vi "svx_SC Line Plot Line Style Write.vi"(4 "error in (no error)":errorcluster, 5 "Value":u8, 6 "Container State":T5, 7 "Display State In":T1={"X Scale"={"Name"="Horizontal", "format string"="%#.2g", "Major Color"=16777238, "Minor Color"=16777216, "Scale Visible"=TRUE, " Label Visible"=TRUE, "Grid Style"=1, "Maximum"=1.0, "Minimum"=-1.0}, "Y Scale"={"Name"="Vertical", "format string"="%#.2g", "Major Color"=16777238, "Minor Color"=16777216, "Scale Visible"=TRUE, " Label Visible"=TRUE, "Grid Style"=1, "Maximum"=1.0, "Minimum"=-1.0}, "Plot"={"Point Style"=0, "Line Width"=0, "Line Style"=0, "Plot Color"=16860, "Point/fill"=16860}, "Arrow Color"=16860, "Autoscale"=TRUE, "Property Name"=[], "Container Bounds"={"Width"=550, "Height"=313}, "Background color"=16777226, "Annotation List"=[], "Cursor"={"Cursor Point Style"=13, "Cursor Style"=4, "Cursor Line Width"=1, "Cursor Line Style"=0, "Cursor Color"=16711680, "Cursor Name Visible"=TRUE, "Cursor Visible"=TRUE, "Cursor Position"={"X"=0.0, "Y"=0.0}, "Cursor Index"=0, "Lock Cursor Name"=FALSE, "Cursor reference"=0.0}, "size"=0, "Boundary Color"=9868950, "Maximum"=1.0, "Marker Point Style"=2, "Maker Visible"=TRUE, "Marker Color"=16860, "pair strings []"=[], "clearance boundary"=[{"boundary"={"x axis"=0.0, "y axis"=0.0}, "start point"=enum."center"}], "Custom pair name"=FALSE, "selector.visible"=TRUE, "Cursor Release"=refnum, "Children Tags"=[], "open?"=TRUE, "pair index"=[], "Legend Width"=200, " Parents Tags"="", "Label"="", "Legend Background"=16777226, "Legend Font"=16777222, "scale fit"=2, "user strings []"=[], "Item Width"=0, "out of state queue"=refnum, "property nodes"=refnum, "Kind"=enum."X-Scale", "Scale Range Change"=refnum} {"pair index" min=0}) -> (0 "error out":errorcluster, 3 "Display State Out":T1={"X Scale"={"Name"="Horizontal", "format string"="%#.2g", "Major Color"=16777238, "Minor Color"=16777216, "Scale Visible"=TRUE, " Label Visible"=TRUE, "Grid Style"=1, "Maximum"=1.0, "Minimum"=-1.0}, "Y Scale"={"Name"="Vertical", "format string"="%#.2g", "Major Color"=16777238, "Minor Color"=16777216, "Scale Visible"=TRUE, " Label Visible"=TRUE, "Grid Style"=1, "Maximum"=1.0, "Minimum"=-1.0}, "Plot"={"Point Style"=0, "Line Width"=0, "Line Style"=0, "Plot Color"=16860, "Point/fill"=16860}, "Arrow Color"=16860, "Autoscale"=TRUE, "Property Name"=[], "Container Bounds"={"Width"=550, "Height"=313}, "Background color"=16777226, "Annotation List"=[], "Cursor"={"Cursor Point Style"=13, "Cursor Style"=4, "Cursor Line Width"=1, "Cursor Line Style"=0, "Cursor Color"=16711680, "Cursor Name Visible"=TRUE, "Cursor Visible"=TRUE, "Cursor Position"={"X"=0.0, "Y"=0.0}, "Cursor Index"=0, "Lock Cursor Name"=FALSE, "Cursor reference"=0.0}, "size"=0, "Boundary Color"=9868950, "Maximum"=1.0, "Marker Point Style"=2, "Maker Visible"=TRUE, "Marker Color"=16860, "pair strings []"=[], "clearance boundary"=[{"boundary"={"x axis"=0.0, "y axis"=0.0}, "start point"=enum."center"}], "Custom pair name"=FALSE, "selector.visible"=TRUE, "Cursor Release"=refnum, "Children Tags"=[], "open?"=TRUE, "pair index"=[], "Legend Width"=200, " Parents Tags"="", "Label"="", "Legend Background"=16777226, "Legend Font"=16777222, "scale fit"=2, "user strings []"=[], "Item Width"=0, "out of state queue"=refnum, "property nodes"=refnum, "Kind"=enum."X-Scale", "Scale Range Change"=refnum} {"pair index" min=0})   [LabVIEW 2017, in "SVX SC Line.xctl"]
uses:
  <vilib>/addons/_XControls/Shaft Centerline/SVX SC Line.xctl
  <vilib>/_xctls/Container State.ctl
  <vilib>/addons/_XControls/Shaft Centerline/subVIs/svx_SC Line State.ctl
  <vilib>/addons/_XControls/Shaft Centerline/subVIs/svx_SC Line Bounds.ctl
  <vilib>/addons/_XControls/Shaft Centerline/subVIs/svx_SC Line Annotation List.ctl
  <vilib>/addons/_XControls/Shaft Centerline/subVIs/svx_SC Line OutState Queue.ctl
  <vilib>/_xctls/XControlSupport.lvlib
panel:
  # "Replace the Value Control below with a Control of desired type.\nDo not remove this Control or the others from the connector pane.\nDo not change the connector pane pattern.\nThe Value control should always be the third terminal from top on the input side in the connector pane."
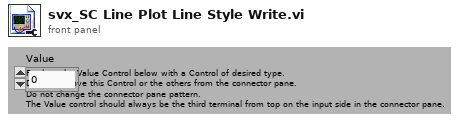
[diagram p1: front panel]
types:
  T1 = typedef "SVX SC Line.xctl/svx_SC Line State.ctl" = cluster{"X Scale":cluster{"Name":string, "format string":string, "Major Color":u32, "Minor Color":u32, "Scale Visible":bool, " Label Visible":bool, "Grid Style":u16, "Maximum":dbl, "Minimum":dbl}, "Y Scale":cluster{"Name":string, "format string":string, "Major Color":u32, "Minor Color":u32, "Scale Visible":bool, " Label Visible":bool, "Grid Style":u16, "Maximum":dbl, "Minimum":dbl}, "Plot":cluster{"Point Style":u8, "Line Width":u8, "Line Style":u8, "Plot Color":u32, "Point/fill":u32}, "Arrow Color":u32, "Autoscale":bool, "Property Name":string[], "Container Bounds":T2, "Background color":u32, "Annotation List":T3, "Cursor":cluster{"Cursor Point Style":u8, "Cursor Style":u8, "Cursor Line Width":u8, "Cursor Line Style":u8, "Cursor Color":u32, "Cursor Name Visible":bool, "Cursor Visible":bool, "Cursor Position":cluster{"X":dbl, "Y":dbl}, "Cursor Index":i32, "Lock Cursor Name":bool, "Cursor reference":dbl}, "size":i32, "Boundary Color":u32, "Maximum":dbl, "Marker Point Style":u8, "Maker Visible":bool, "Marker Color":u32, "pair strings []":string[], "clearance boundary":cluster{"boundary":cluster{"x axis":dbl, "y axis":dbl}, "start point":enum16{"center", "top", "bottom"}}[], "Custom pair name":bool, "selector.visible":bool, "Cursor Release":refnum<user-event>, "Children Tags":string[], "open?":bool, "pair index":i32[], "Legend Width":u32, " Parents Tags":string, "Label":string, "Legend Background":u32, "Legend Font":u32, "scale fit":u8, "user strings []":string[], "Item Width":u32, "out of state queue":T4, "property nodes":refnum<queue>, "Kind":enum16{"X-Scale", "Y-Scale", "Z-Scale"}, "Scale Range Change":refnum<user-event>}
  T2 = typedef "SVX SC Line.xctl/svx_SC Line Bounds.ctl" = cluster{"Width":u32, "Height":u32}
  T3 = typedef "SVX SC Line.xctl/svx_SC Line Annotation List.ctl" = cluster{"Name":string, "Color":u32, "Style":u8, "Point Style":u8, "Name Visible":bool, "Allow Drag":bool, "Annotation Mode":u32, "Plot":i32, "Index":i32, "Position":cluster{"X":dbl, "Y":dbl}, "X Scale":u32, "Y Scale":u32, "Show Arrow":bool, "Lock Name":bool, "Plot Area":i32, "Label Offset":cluster{"X":dbl, "Y":dbl}}[]
  T4 = typedef "SVX SC Line.xctl/svx_SC Line OutState Queue.ctl" = refnum<queue>
  T5 = typedef "XControlSupport.lvlib/Container State.ctl" = cluster{"Indicator?":bool, "Run Mode?":bool, " Refnum":refnum<vi>}
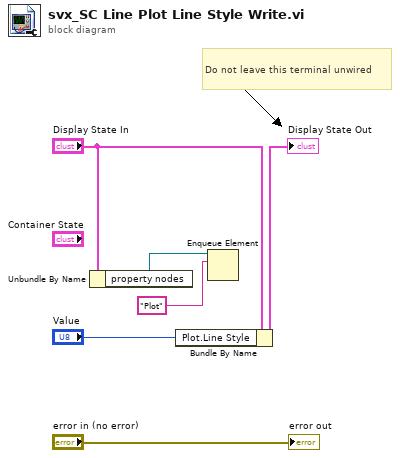
[diagram p0: block diagram]
diagram:
  # "Do not leave this terminal unwired"
  n1 = Unbundle By Name("Display State In") -> ("property nodes"=w2:refnum<queue>)
  n2 = Bundle By Name(cluster="Display State In", "Plot.Line Style"="Value") -> (→"Display State Out":T1)
  n3 = Enqueue Element(queue=w2, element="Plot" ("Property Name")) -> ()  [unwired: 2 in, 3 out]
  "error out" <- "error in (no error)"
